vi "Shut Down Device.vi"(8 "error in (no error)":errorcluster, 11 "Orca-Flash 4.0 in":refnum<class "Hamamatsu Camera.lvclass">) -> (0 "error out":errorcluster, 3 "Orca-Flash 4.0 out":refnum<class "Hamamatsu Camera.lvclass">)   [LabVIEW 2018, in "Hamamatsu Camera.lvlib" / "Hamamatsu Camera.lvclass"]
uses:
  Hamamatsu Camera.lvclass
  Camera/Camera.lvclass
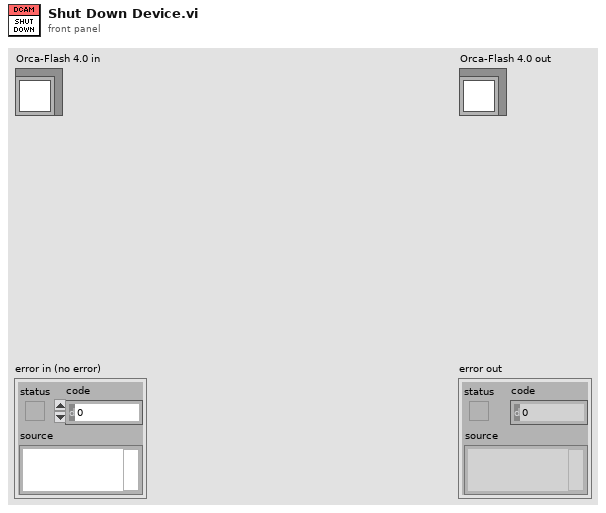
[diagram p1: front panel]
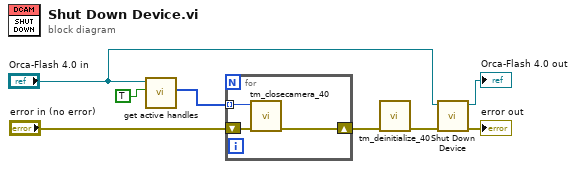
[diagram p0: block diagram]
diagram:
  n1 = call-dynamic "get active handles.vi"("Return All?"=TRUE, "Camera in"="Orca-Flash 4.0 in") -> ("Handles"=w2:u32[])  [unwired: 5 in, 4 out]
  n2 = for {
    tunnel: w2 -> [w10] mode=indexing
    shift-right: [w9] -> w5
    shift-left: "error in (no error)" -> [w11]
    n3 = call <userlib>:"tm_closecamera_40.vi"("error in (no error)"=w11, "Handle in"=w10) -> ("error out"=w9:errorcluster)  [unwired: 9 in]
  }
  n4 = call <userlib>:"tm_deinitialize_40.vi"("error in (no error)"=w5) -> ("error out"=w4:errorcluster)  [unwired: 10 in]
  n5 = call-parent "Shut Down Device.vi"("error in (no error)"=w4, "Device in"="Orca-Flash 4.0 in") -> ("error out"=→"error out":errorcluster, "Device out"=→"Orca-Flash 4.0 out":refnum<class "Hamamatsu Camera.lvclass">)  [unwired: 8 in]
